vi "workspace.get_all.vi"(8 "error in":errorcluster, 11 "Nominal Client in":refnum<class "Nominal Client.lvclass">) -> (0 "error out":errorcluster, 2 "Workspaces":T1(array[cluster]), 3 "Nominal Client out":refnum<class "Nominal Client.lvclass">)   [LabVIEW 2020, in "Nominal Client.lvclass"]
doc: "Gets all workspaces that the requesting user belongs to."
uses:
  Nominal Client.lvclass
  ce527530-f409-488f-b07f-3b5ecba8805e.vi
  <vilib>/JDP Science/JSONtext/JSON text to Variant.vi
  <vilib>/JDP Science/JSONtext/LVClass Serializer/JSONtext LVClass Serializer.lvclass
  Nominal Client.lvclass/Nominal Client.ctl
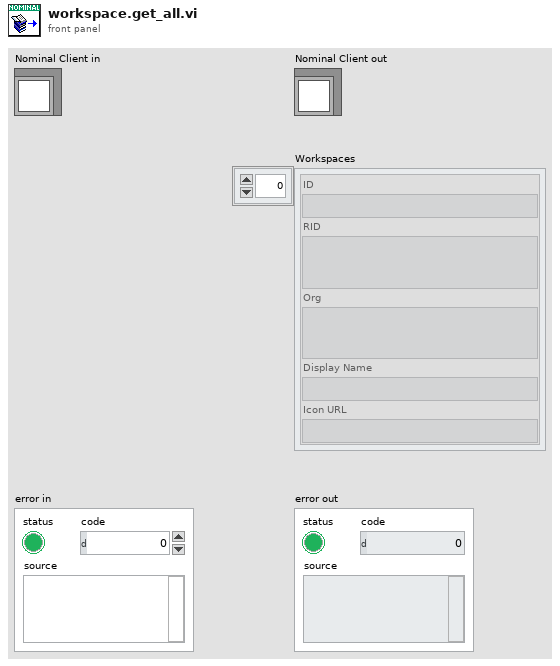
[diagram p1: front panel]
types:
  T1 = cluster{"ID":string, "RID":string, "Org":string, "Display Name":string, "Icon URL":string}[]
  T2 = cluster{"id":string, "rid":string, "org":string, "displayName":string, "iconUrl":string}[]
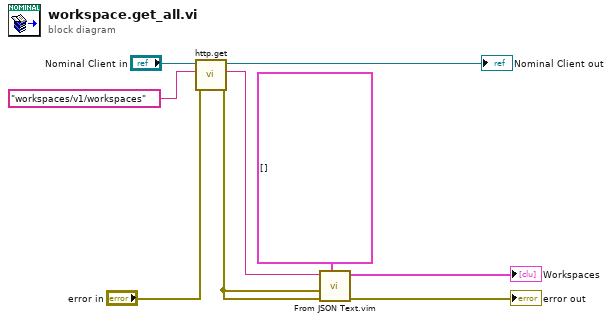
[diagram p0: block diagram]
diagram:
  n1 = call "http.get.vi"("error in"="error in", "Path"="workspaces/v1/workspaces", "Nominal Client in"="Nominal Client in") -> ("error out"=w1:errorcluster, "Response"=w4:string, "Nominal Client out"=→"Nominal Client out":refnum<class "Nominal Client.lvclass">)  [unwired: 5 in, 1 out]
  "error out" <- w1
  n2 = call "From JSON Text.vim"("Data Type and Default Value"=T2 [] ("Workspaces"), "error in (no error)"=w1, "JSON"=w4) -> ("Data out"=→"Workspaces":T2)  [unwired: 7 in, 1 out]
